vi "Waveform Analysis (Polling).vi"() -> ()   [LabVIEW 2012]
uses:
  <vilib>/Analysis/NI_AALPro.lvlib
  <vilib>/Analysis/2dsp.llb/Real FFT.vi
panel:
  out "Spectrum":dbl[](graph)
  out "Min":dbl
  out "Max":dbl
  out "Time Series":dbl[](graph)
  in  "Get Max & Min":bool
  in  "Calculate FFT":bool
  in  "Get Time Series":bool
  in  "Stop":bool
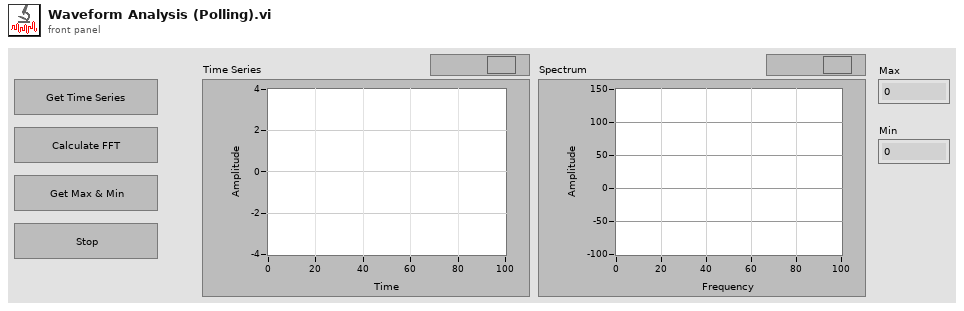
[diagram p1: front panel]
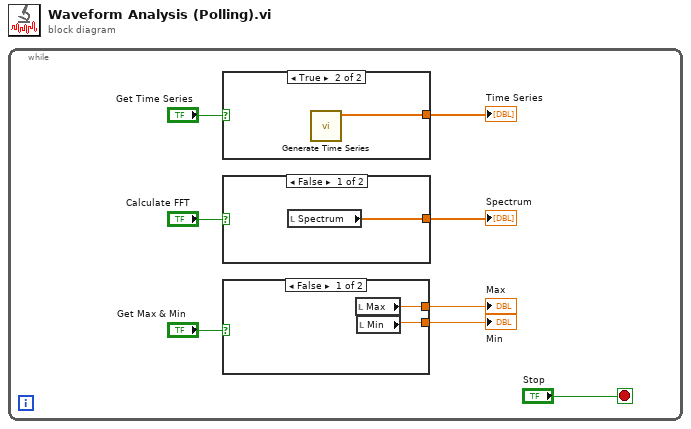
[diagram p0: block diagram]
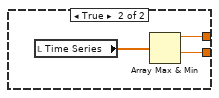
[diagram p2: hidden frame]
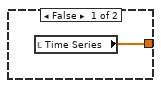
[diagram p3: hidden frame]
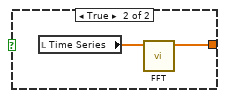
[diagram p4: hidden frame]
diagram:
  n1 = while {
    stop <- "Stop" stop-if-true
    n2 = case shown="True" "Get Time Series" {
      tunnel: [w14 w15] -> w4
      frame False {
        n3 = local read "Time Series"() -> (w14:dbl[])
      }
      frame True {
        n4 = call "Generate Time Series.vi"() -> ("Time Series"=w15:dbl[])  [unwired: 11 in]
      }
    }
    "Time Series" <- w4
    n5 = case shown="False" "Calculate FFT" {
      tunnel: [w16 w17] -> w1
      frame False {
        n6 = local read "Spectrum"() -> (w16:dbl[])
      }
      frame True {
        n7 = local read "Time Series"() -> (w18:dbl[])
        n8 = call-poly <vilib>:"FFT.vi"("X"=w18) -> ("FFT {X}"=w17:cdb[])  [unwired: 9 in, 1 out]
      }
    }
    "Spectrum" <- w1
    n9 = case shown="False" "Get Max & Min" {
      tunnel: [w10 w12] -> w3
      tunnel: [w9 w11] -> w2
      frame False {
        n10 = local read "Max"() -> (w10:dbl)
        n11 = local read "Min"() -> (w9:dbl)
      }
      frame True {
        n12 = local read "Time Series"() -> (w13:dbl[])
        n13 = Array Max & Min(array=w13) -> (max value=w12:dbl, min value=w11:dbl)  [unwired: 2 out]
      }
    }
    "Max" <- w3
    "Min" <- w2
  }
